vi "Create Serial Output Channel Mask.vi"(0 "serial channels":string[](array[string])) -> (4 "serial output channel mask":bool[](array[boolean]))   [LabVIEW 2023, in "GettingStarted_Gen_148X_Host.lvlib"]
uses:
  GettingStarted_Gen_148X_Host.lvlib
  <instrlib>/FlexRIO/Automotive Vision Utility/v1/Host/Automotive Vision Utility.lvlib
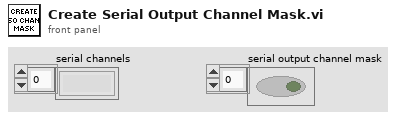
[diagram p1: front panel]
types:
  T1 = typedef "Automotive Vision Utility.lvlib/Serial Channel Type.ctl" = enum16{"Serial Input Channel", "Serial Output Channel", "Unknown Channel Type"}
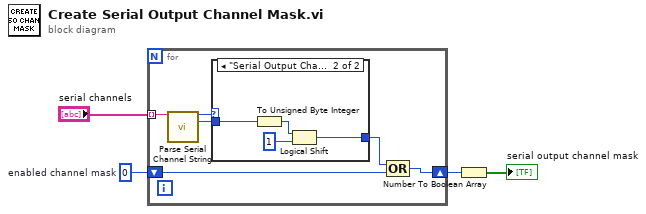
[diagram p0: block diagram]
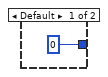
[diagram p2: hidden frame]
diagram:
  w2 = u8 0  # enabled channel mask
  n1 = for {
    tunnel: "serial channels" -> [w10] mode=indexing
    shift-right: [w6] -> w3
    shift-left: w2 -> [w5]
    n2 = call <instrlib>:"Parse Serial Channel String.vi"("serial channel string"=w10) -> ("serial channel type"=w9:T1, "channel number"=w8:i32)  [unwired: 13 in]
    n3 = case shown="\"Serial Output Channel\"" w9 {
      tunnel: w8 -> [_ w14]
      tunnel: [u8 0 w12] -> w7
      frame Default {
      }
      frame "Serial Output Channel" {
        n4 = To Unsigned Byte Integer(number=w14) -> (unsigned 8bit integer=w13:u8)
        n5 = Logical Shift(y=w13, x=u8 1) -> (x << y=w12:u8)
      }
    }
    n6 = Compound Arithmetic op=OR(w7, w5) -> (w6:u8)
  }
  n7 = Number To Boolean Array(number=w3) -> (Boolean array=→"serial output channel mask":bool[])
